vi "Read Event Name.vi"(8 "error in (no error)":errorcluster, 11 "TAS_Event in":refnum<class "TAS_Event.lvclass">) -> (0 "error out":errorcluster, 2 "Event Name":string, 3 "TAS_Event out":refnum<class "TAS_Event.lvclass">)   [LabVIEW 2012, in "TAS_Event.lvclass"]
uses:
  TAS_Event.lvclass
  TAS_Event.lvclass/TAS_Event.ctl
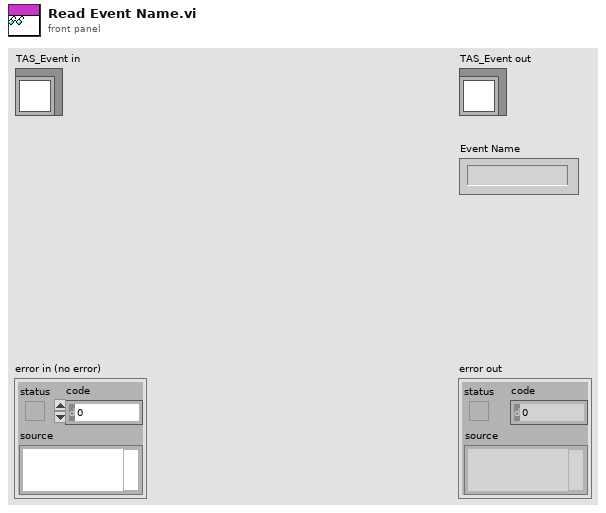
[diagram p1: front panel]
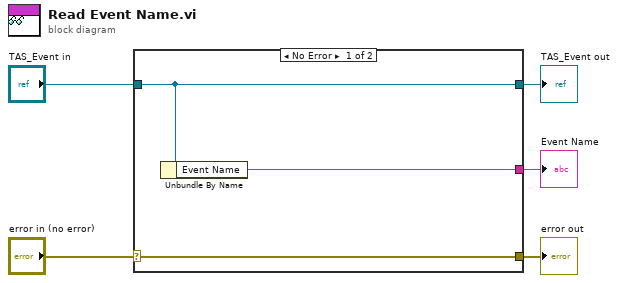
[diagram p0: block diagram]
diagram:
  n1 = case shown="No Error" "error in (no error)" {
    selector: "error in (no error)" -> [w8 w9]
    tunnel: [w8 w9] -> w4
    tunnel: [w7 w10] -> w2
    tunnel: "TAS_Event in" -> [w7 w10]
    tunnel: [w6 _] -> w1
    frame No Error {
      n2 = Unbundle By Name(w7) -> ("Event Name"=w6:string)
    }
    frame Error {
    }
  }
  "error out" <- w4
  "TAS_Event out" <- w2
  "Event Name" <- w1
